vi "Write New Class Path.vi"(8 "error in (no error)":errorcluster, 10 "New Class Path":path, 11 "New QControl Info in":refnum<class "New QControl Info.lvclass">) -> (0 "error out":errorcluster, 3 "New QControl Info out":refnum<class "New QControl Info.lvclass">)   [LabVIEW 2015, in "New QControl Info.lvclass"]
uses:
  New QControl Info.lvclass
  New QControl Info.lvclass/New QControl Info.ctl
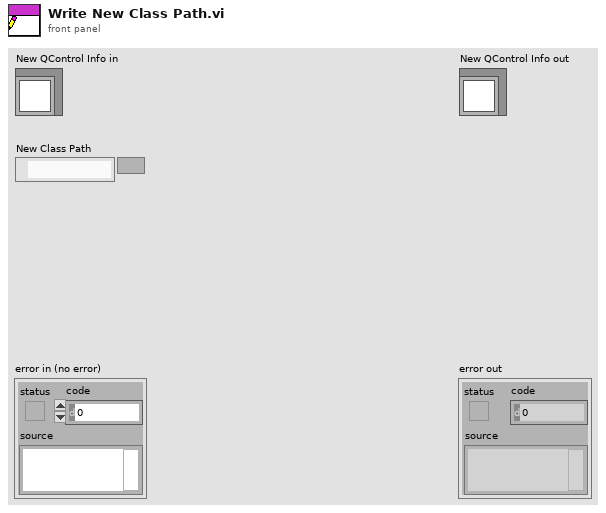
[diagram p1: front panel]
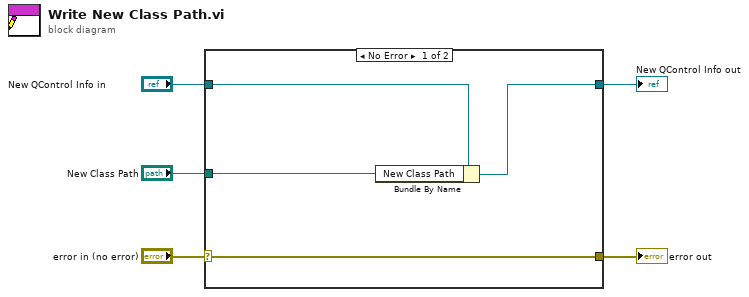
[diagram p0: block diagram]
diagram:
  n1 = case shown="No Error" "error in (no error)" {
    selector: "error in (no error)" -> [w9 w10]
    tunnel: [w9 w10] -> w4
    tunnel: [w7 w11] -> w2
    tunnel: "New QControl Info in" -> [w8 w11]
    tunnel: "New Class Path" -> [w6 _]
    frame No Error {
      n2 = Bundle By Name(cluster=w8, "New Class Path"=w6) -> (w7:refnum<class "New QControl Info.lvclass">)
    }
    frame Error {
    }
  }
  "error out" <- w4
  "New QControl Info out" <- w2
